vi "OSCILO_W_HEADER.vi"(0 "TCP Network Connection in":refnum<k5>, 1 "TRIGGER_LEVEL":u32, 3 "FIFO_SIZE":u32, 5 "dt (ns)":u32, 9 "TRIG_DELAY":u32, 11 "error in (no error)":errorcluster, 12 "SET":bool, 14 "Trigger Edge":u32) -> (4 "TCP Network Connection out":refnum<k5>, 6 "output waveform":waveform(dbl), 8 "Timestamp":u64 format="%.0x", 10 "DATA_AVAILABLE":bool, 15 "error out":errorcluster)   [LabVIEW 2019]
panel:
  out "x-y":dbl
  out "time stamp":timestamp
  out "Event_number":u8
  out "TAIL":u32[](array[numeric]) format="%.0x"
  out "HEAD":u32[](array[numeric]) format="%.0x"
  out "Oscilloscope":u32[](array[numeric])
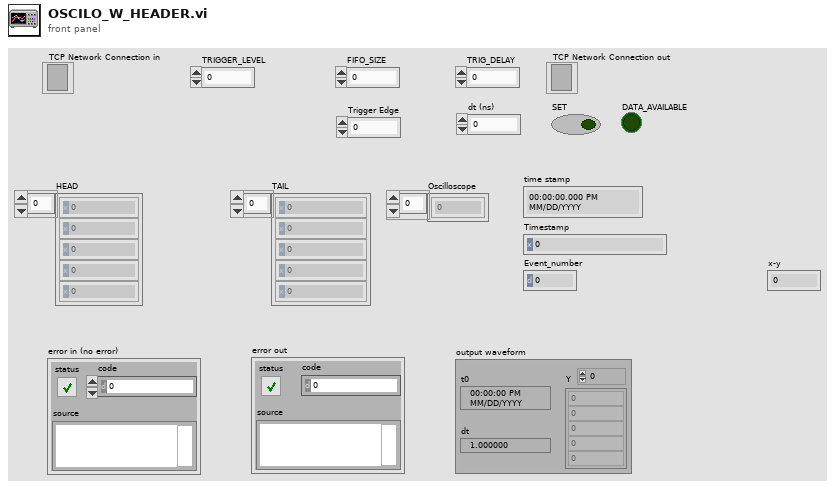
[diagram p1: front panel]
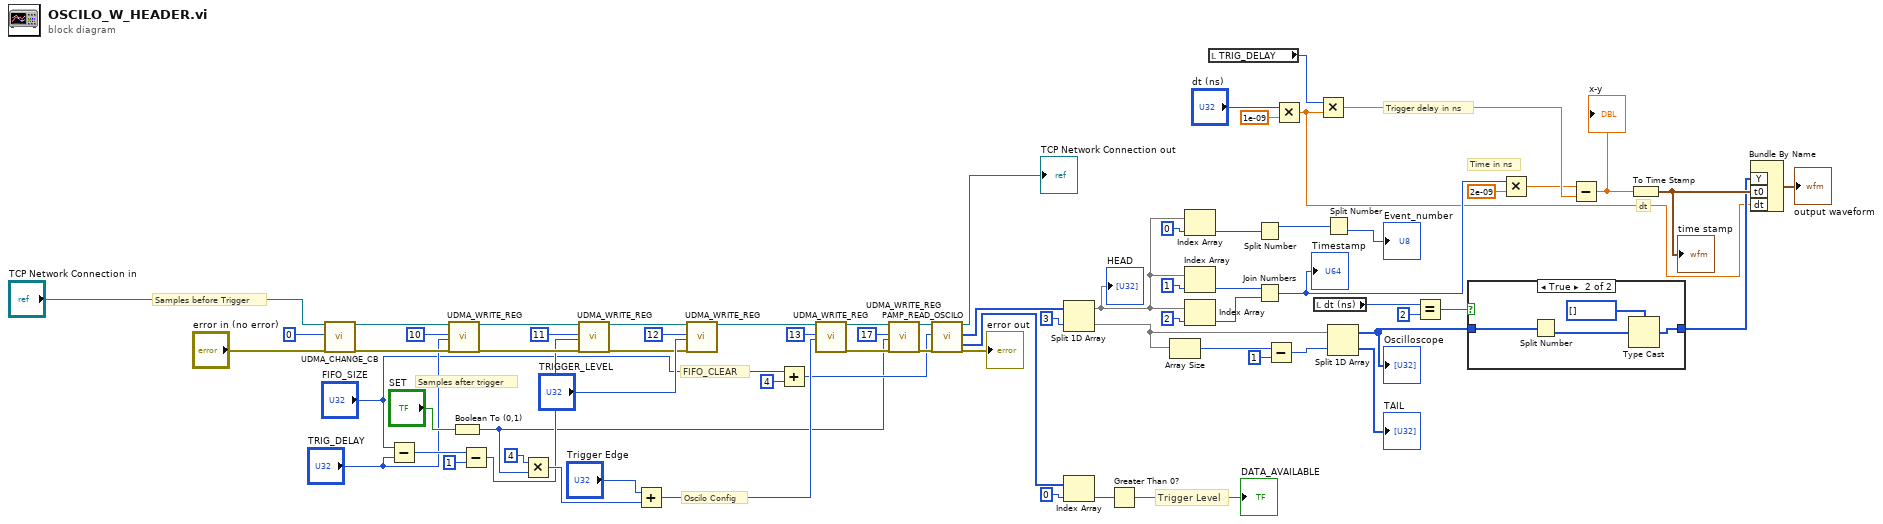
[diagram p0: block diagram]
diagram:
  # "Trigger delay in ns"
  # "dt"
  # "Time in ns"
  # "FIFO_CLEAR"
  # "Oscilo Config"
  # "Trigger Level"
  # "Samples after trigger"
  # "Samples before Trigger"
  n1 = call "UDMA_CHANGE_CB.vi"("TCP Network Connection in"="TCP Network Connection in", "CB_ID"=u32 0, "error in (no error)"="error in (no error)") -> ("TCP Network Connection out"=w44:refnum<k5>, "error out"=w43:errorcluster)  [unwired: 14 in, 1 out]
  n2 = Subtract(x="FIFO_SIZE", y="TRIG_DELAY") -> (x-y=w61:u32)
  n3 = call "UDMA_WRITE_REG.vi"("TCP Network Connection in"=w44, "REG"=u32 10, "DATA"="TRIG_DELAY", "error in (no error)"=w43) -> ("TCP Network Connection out"=w63:refnum<k5>, "error out"=w62:errorcluster)  [unwired: 13 in, 1 out]
  n4 = Boolean To (0,1)(Boolean="SET") -> (0, 1=w1:i16)
  n5 = Subtract(x=w61, y=u32 1) -> (x-y=w60:u32)
  n6 = Multiply(x=i16 4, y=w1) -> (x*y=w64:i16)
  n7 = call "UDMA_WRITE_REG.vi"("TCP Network Connection in"=w63, "REG"=u32 11, "DATA"=w60, "error in (no error)"=w62) -> ("TCP Network Connection out"=w55:refnum<k5>, "error out"=w54:errorcluster)  [unwired: 13 in, 1 out]
  n8 = Add(x="Trigger Edge", y=w64) -> (x+y=w58:u32)
  n9 = call "UDMA_WRITE_REG.vi"("TCP Network Connection in"=w55, "REG"=u32 12, "DATA"="TRIGGER_LEVEL", "error in (no error)"=w54) -> ("TCP Network Connection out"=w56:refnum<k5>)  [unwired: 13 in, 2 out]
  n10 = Add(x="FIFO_SIZE", y=u32 4) -> (x+y=w11:u32)
  n11 = call "UDMA_WRITE_REG.vi"("TCP Network Connection in"=w56, "REG"=u32 13, "DATA"=w58) -> ("TCP Network Connection out"=w51:refnum<k5>, "error out"=w52:errorcluster)  [unwired: 14 in, 1 out]
  n12 = call "UDMA_WRITE_REG.vi"("TCP Network Connection in"=w51, "REG"=u32 17, "DATA"=w1, "error in (no error)"=w52) -> ("TCP Network Connection out"=w13:refnum<k5>, "error out"=w12:errorcluster)  [unwired: 13 in, 1 out]
  n13 = call "PAMP_READ_OSCILO.vi"("TCP Network Connection in"=w13, "N"=w11, "error in (no error)"=w12) -> ("TCP Network Connection out"=→"TCP Network Connection out":refnum<k5>, "Oscilloscope"=w3:u32[], "Status"=w8:u8[], "error out"=→"error out":errorcluster)  [unwired: 12 in, 1 out]
  n14 = Split 1D Array(array=w3, index=3) -> (first subarray=w32:u32[], second subarray=w7:u32[])
  "HEAD" <- w32
  n15 = Index Array(array=w8, index=0) -> (element=w48:u8)
  n16 = Greater Than 0?(x=w48) -> (x > 0?=→"DATA_AVAILABLE":bool)
  n17 = Array Size(array=w7) -> (size(s)=w6:i32)
  n18 = Index Array(array=w32, index=0) -> (element=w31:u32)
  n19 = Index Array(array=w32, index=1) -> (element=w35:u32)
  n20 = Index Array(array=w32, index=2) -> (element=w34:u32)
  n21 = local read "TRIG_DELAY"() -> (w17:u32)
  n22 = Split Number(x=w31) -> (hi(x)=w30:u16)  [unwired: 1 out]
  n23 = Join Numbers(hi=w35, lo=w34) -> ((hi.lo)=w20:u64)
  "Timestamp" <- w20
  n24 = Subtract(x=w6, y=1) -> (x-y=w4:i32)
  n25 = Multiply(x="dt (ns)", y=1e-09) -> (x*y=w18:dbl)
  n26 = local read "dt (ns)"() -> (w25:u32)
  n27 = Multiply(x=w17, y=w18) -> (x*y=w16:dbl)
  n28 = Split Number(x=w30) -> (lo(x)=→"Event_number":u8)  [unwired: 1 out]
  n29 = Split 1D Array(array=w7, index=w4) -> (first subarray=w22:u32[], second subarray=→"TAIL":u32[])
  "Oscilloscope" <- w22
  n30 = Equal?(x=w25, y=u32 2) -> (x = y?=w23:bool)
  n31 = case shown="True" w23 {
    tunnel: [w72 w75] -> w21
    tunnel: w22 -> [w72 w74]
    frame False {
    }
    frame True {
      n32 = Split Number(x=w74) -> (lo(x)=w73:u16[])  [unwired: 1 out]
      n33 = Type Cast(type=u8[] [] ("Oscilloscope"), x=w73) -> (*(type *) &x=w75:u8[])
    }
  }
  n34 = Multiply(x=w20, y=2e-09) -> (x*y=w15:dbl)
  n35 = Subtract(x=w15, y=w16) -> (x-y=w14:dbl)
  "x-y" <- w14
  n36 = To Time Stamp(1:w14) -> (0:w26:timestamp)
  "time stamp" <- w26
  n37 = Bundle By Name("Y"=w21, "t0"=w26, "dt"=w18) -> (→"output waveform":waveform(u32))  [unwired: 1 in]
